vi "Get Frequency List - NF.vi"(11 "UI Controls":T3 {"measurement configuration"."Noise Source Loss S-Parameter Orientation" items=["Port1 Towards DUT", "Port2 Towards DUT"]; "measurement configuration"."Calibration Loss S-Parameter Orientation" items=["Port1 Towards DUT", "Port2 Towards DUT"]; "measurement configuration"."DUT Output Loss S-Parameter Orientation" items=["Port1 Towards DUT", "Port2 Towards DUT"]; "measurement configuration"."DUT Input Loss S-Parameter Orientation" items=["Port1 Towards DUT", "Port2 Towards DUT"]; "measurement configuration"."FreqList - Frequency List" format="%.3p Hz"; "measurement configuration"."Points - Stop Frequency" format="%.3p Hz"; "measurement configuration"."Points - Start Frequency" format="%.3p Hz"; "measurement configuration"."Step - Step Size" format="%.3p Hz"; "measurement configuration"."Step - Stop Frequency" format="%.3p Hz"; "measurement configuration"."Step - Start Frequency" format="%.3p Hz"; "measurement configuration"."Noise Source_Loss (dB)" format="%.2g"; "measurement configuration"."Noise Source_Loss Freq (Hz)" format="%.3p"; "measurement configuration"."Noise Source_Temperation (K)" format="%.2g"; "measurement configuration"."Calibration_Loss (dB)" format="%.2g"; "measurement configuration"."Calibration_Loss Freq (Hz)" format="%.3p"; "measurement configuration"."Calibration_Temperation (K)" format="%.2g"; "measurement configuration"."DUT Output_Loss (dB)" format="%.2g"; "measurement configuration"."DUT Output_Loss Freq (Hz)" format="%.3p"; "measurement configuration"."DUT Output_Temperation (K)" format="%.2g"; "measurement configuration"."DUT Input_Loss (dB)" format="%.2g"; "measurement configuration"."DUT Input_Loss Freq (Hz)" format="%.3p"; "measurement configuration"."DUT Input_Temperation (K)" format="%.2g"; "measurement configuration"."ENR (dB)" format="%.2g"; "measurement configuration"."ENR Freq (Hz)" format="%.3p"; "measurement configuration"."Noise Source Off Temperature (K)" format="%.2f"; "measurement configuration"."Noise Source Cold Temperature (K)" format="%.2f"; "measurement configuration"."Noise Source Type" items=["External Noise Source", "RF Signal Generator"]; "measurement configuration"."DUT Type" items=["Amplifier", "Downconverter", "Upconverter"]; "measurement configuration"."Measurement Interval (s)" format="%.2p"; "measurement configuration"."Measurement Bandwidth (Hz)" format="%.3p"; "measurement configuration"."Action" items=["Measure", "Calibrate"]; "measurement configuration"."RFmx external attenuation (dB)" format="%.2f"; "measurement configuration"."Preamp Enabled" items=["Disabled"=0, "Enabled"=1, "Automatic"=3]; "measurement results"."Analyzer NF (mean)" format="%.2g"; "measurement results"."DUT NF (mean)" format="%.2g"; "measurement results"."Analyzer NF vs Freq" format="%.2g"; "measurement results"."DUT NF vs Freq" format="%.2g"}) -> (3 "Frequency List":dbl[](array[numeric]) format="%.3p Hz")   [LabVIEW 2023, in "FPT NoiseFigure.lvclass"]
uses:
  FPT NoiseFigure.lvclass
  Measurement Configuration.ctl
  Measurement Results.ctl
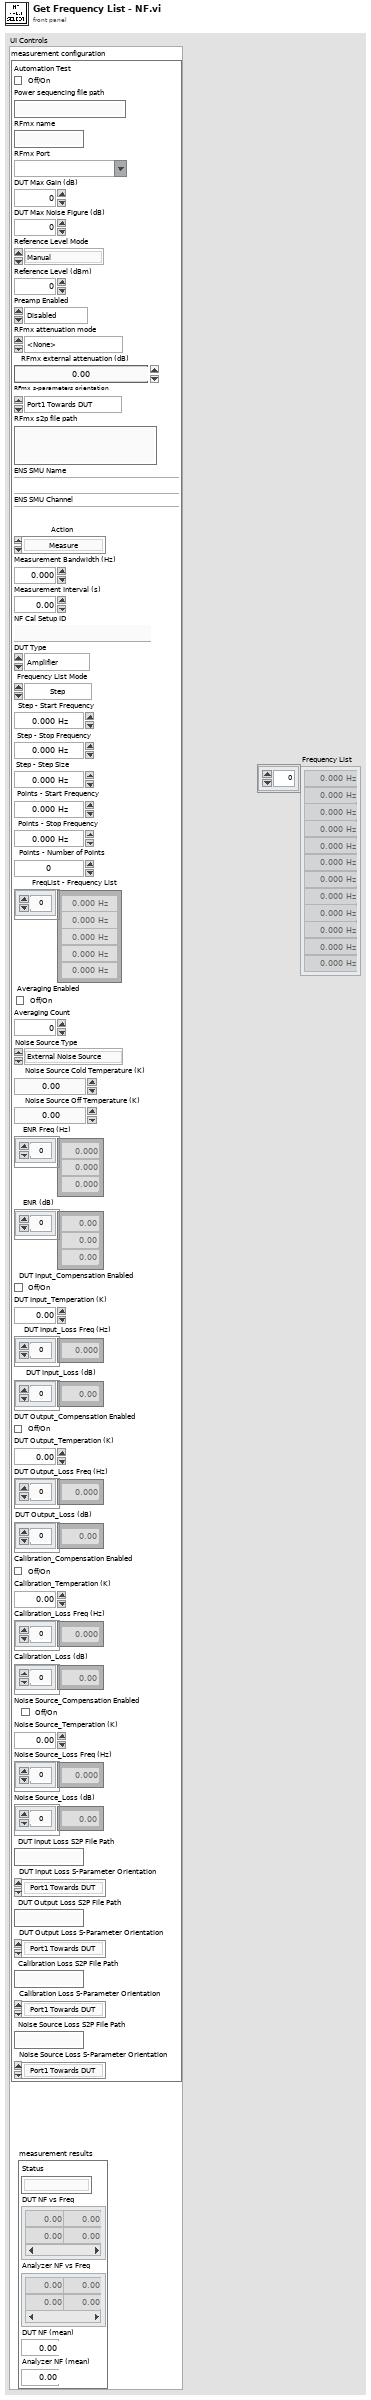
[diagram p1: front panel]
types:
  T1 = typedef "FPT NoiseFigure.lvclass/Measurement Configuration.ctl" = cluster{"Automation Test":bool, "Power sequencing file path":string, "RFmx name":string, "RFmx port":string, "DUT Max Gain (dB)":dbl, "DUT Max Noise Figure (dB)":dbl, "Reference Level Mode":enum32{"Manual", "Recommend"}, "Reference Level (dBm)":dbl, "Preamp Enabled":i32, "RFmx attenuation mode":enum32{"<None>", "Constant Attenuation", "s2p File"}, "RFmx external attenuation (dB)":dbl, "RFmx s-parameters orientation":enum32{"Port1 Towards DUT", "Port2 Towards DUT"}, "RFmx s2p file path":string, "ENS SMU Name":string, "ENS SMU Channel":string, "Action":u32, "Measurement Bandwidth (Hz)":dbl, "Measurement Interval (s)":dbl, "NF Cal Setup ID":string, "DUT Type":i32, "Frequency List Mode":enum32{"Step", "Points", "Frequency List"}, "Step - Start Frequency ":dbl, "Step - Stop Frequency":dbl, "Step - Step Size":dbl, "Points - Start Frequency":dbl, "Points - Stop Frequency":dbl, "Points - Number of Points":i32, "FreqList - Frequency List":dbl[], "Averaging Enabled":bool, "Averaging Count":i32, "Noise Source Type":i32, "Noise Source Cold Temperature (K)":dbl, "Noise Source Off Temperature (K)":dbl, "ENR Freq (Hz)":dbl[], "ENR (dB)":dbl[], "DUT Input_Compensation Enabled":bool, "DUT Input_Temperation (K)":dbl, "DUT Input_Loss Freq (Hz)":dbl[], "DUT Input_Loss (dB)":dbl[], "DUT Output_Compensation Enabled":bool, "DUT Output_Temperation (K)":dbl, "DUT Output_Loss Freq (Hz)":dbl[], "DUT Output_Loss (dB)":dbl[], "Calibration_Compensation Enabled":bool, "Calibration_Temperation (K)":dbl, "Calibration_Loss Freq (Hz)":dbl[], "Calibration_Loss (dB)":dbl[], "Noise Source_Compensation Enabled":bool, "Noise Source_Temperation (K)":dbl, "Noise Source_Loss Freq (Hz)":dbl[], "Noise Source_Loss (dB)":dbl[], "DUT Input Loss S2P File Path":string, "DUT Input Loss S-Parameter Orientation":i32, "DUT Output Loss S2P File Path":string, "DUT Output Loss S-Parameter Orientation":i32, "Calibration Loss S2P File Path":string, "Calibration Loss S-Parameter Orientation":i32, "Noise Source Loss S2P File Path":string, "Noise Source Loss S-Parameter Orientation":i32}
  T2 = typedef "FPT NoiseFigure.lvclass/Measurement Results.ctl" = cluster{"Status":string, "DUT NF vs Freq":dbl[][], "Analyzer NF vs Freq":dbl[][], "DUT NF (mean)":dbl, "Analyzer NF (mean)":dbl}
  T3 = cluster{"measurement configuration":T1, "measurement results":T2}
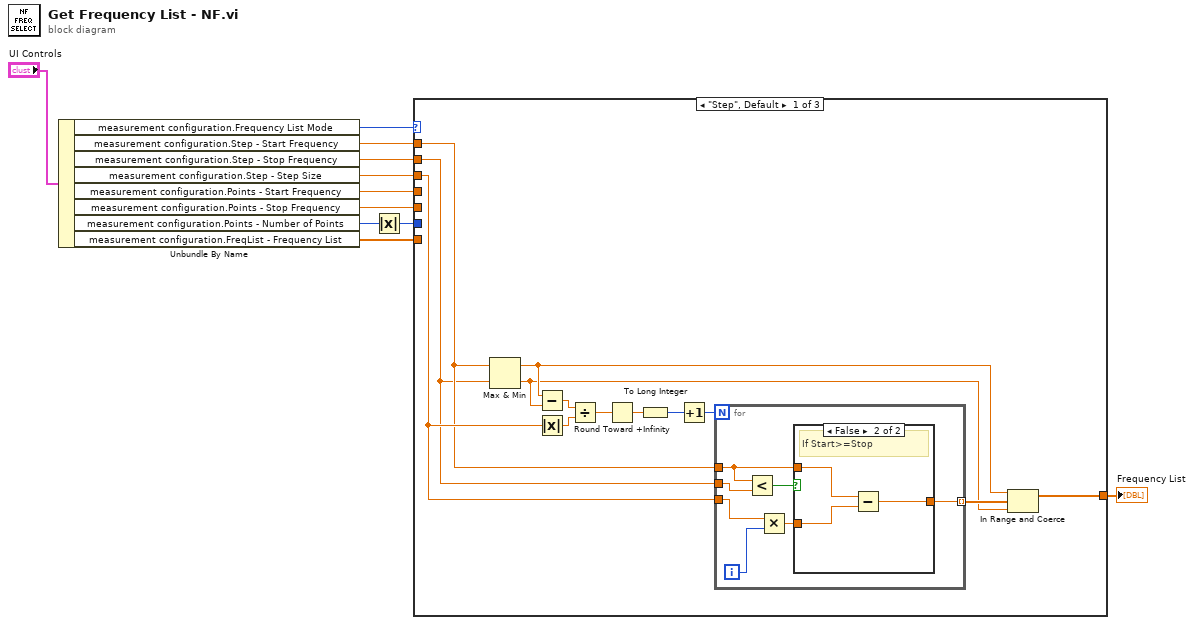
[diagram p0: block diagram]
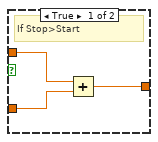
[diagram p2: hidden frame]
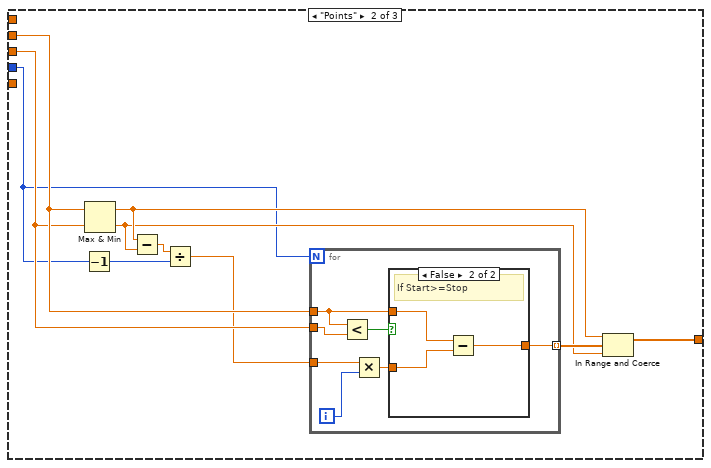
[diagram p3: hidden frame]
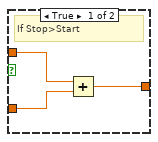
[diagram p4: hidden frame]
diagram:
  n1 = Unbundle By Name("UI Controls") -> ("measurement configuration.Frequency List Mode"=w1:enum32{"Step", "Points", "Frequency List"}, "measurement configuration.Step - Start Frequency"=w10:dbl, "measurement configuration.Step - Stop Frequency"=w9:dbl, "measurement configuration.Step - Step Size"=w8:dbl, "measurement configuration.Points - Start Frequency"=w6:dbl, "measurement configuration.Points - Stop Frequency"=w5:dbl, "measurement configuration.Points - Number of Points"=w4:i32, "measurement configuration.FreqList - Frequency List"=w3:dbl[])
  n2 = Absolute Value(x=w4) -> (abs(x)=w2:i32)
  n3 = case shown="\"Step\", Default" w1 {
    tunnel: w10 -> [w19 _ _]
    tunnel: w9 -> [w18 _ _]
    tunnel: w8 -> [w21 _ _]
    tunnel: [w14 w43 w61] -> w7
    tunnel: w6 -> [_ w42 _]
    tunnel: w5 -> [_ w41 _]
    tunnel: w2 -> [_ w40 _]
    tunnel: w3 -> [_ _ w61]
    frame "Step", Default {
      n4 = Max & Min(x=w19, y=w18) -> (max(x,y)=w16:dbl, min(x,y)=w15:dbl)
      n5 = Subtract(x=w16, y=w15) -> (x-y=w17:dbl)
      n6 = Absolute Value(x=w21) -> (abs(x)=w24:dbl)
      n7 = Divide(x=w17, y=w24) -> (x/y=w23:dbl)
      n8 = Round Toward +Infinity(x=w23) -> (ceil(x): smallest int >= x=w12:dbl)
      n9 = To Long Integer(number=w12) -> (32bit integer=w22:i32)
      n10 = Increment(x=w22) -> (x+1=w13:i32)
      n11 = for {
        N: w13 -> [_]
        tunnel: w19 -> [w27]
        tunnel: w18 -> [w26]
        tunnel: w21 -> [w31]
        tunnel: [w25] -> w20 mode=indexing
        i -> [w30]
        n12 = Less?(x=w27, y=w26) -> (x < y?=w28:bool)
        n13 = Multiply(x=w31, y=w30) -> (x*y=w29:dbl)
        n14 = case shown="False" w28 {
          tunnel: w27 -> [w34 w37]
          tunnel: w29 -> [w33 w36]
          tunnel: [w32 w35] -> w25
          frame True {
            # "If Stop>Start"
            n15 = Add(x=w34, y=w33) -> (x+y=w32:dbl)
          }
          frame False {
            # "If Start>=Stop"
            n16 = Subtract(x=w37, y=w36) -> (x-y=w35:dbl)
          }
        }
      }
      n17 = In Range and Coerce(upper limit=w16, x=w20, lower limit=w15) -> (coerced(x)=w14:dbl[])  [unwired: 1 out]
    }
    frame "Points" {
      n18 = Decrement(x=w40) -> (x-1=w38:i32)
      n19 = Max & Min(x=w42, y=w41) -> (max(x,y)=w45:dbl, min(x,y)=w44:dbl)
      n20 = Subtract(x=w45, y=w44) -> (x-y=w46:dbl)
      n21 = Divide(x=w46, y=w38) -> (x/y=w39:dbl)
      n22 = for {
        N: w40 -> [_]
        tunnel: w42 -> [w51]
        tunnel: w41 -> [w50]
        tunnel: [w49] -> w47 mode=indexing
        tunnel: w39 -> [w48]
        i -> [w54]
        n23 = Less?(x=w51, y=w50) -> (x < y?=w52:bool)
        n24 = Multiply(x=w48, y=w54) -> (x*y=w53:dbl)
        n25 = case shown="False" w52 {
          tunnel: w51 -> [w57 w60]
          tunnel: w53 -> [w56 w59]
          tunnel: [w55 w58] -> w49
          frame True {
            # "If Stop>Start"
            n26 = Add(x=w57, y=w56) -> (x+y=w55:dbl)
          }
          frame False {
            # "If Start>=Stop"
            n27 = Subtract(x=w60, y=w59) -> (x-y=w58:dbl)
          }
        }
      }
      n28 = In Range and Coerce(upper limit=w45, x=w47, lower limit=w44) -> (coerced(x)=w43:dbl[])  [unwired: 1 out]
    }
    frame "Frequency List" {
    }
  }
  "Frequency List" <- w7
